vi "aotfController.vi"() -> ()   [LabVIEW 2024]
uses:
  <vilib>/Utility/error.llb/Trim Whitespace One-Sided.vi
  <vilib>/Instr/_visa.llb/VISA Configure Serial Port (Instr).vi
panel:
  in  "Stop Button":bool
  in  "Use":bool
  out "myaotf":refnum<k38>
  out "VISA out":refnum<visa-resource-name>="COM7"
  in  "VISA resource name":refnum<visa-resource-name>="COM7"
  out "module path":path=path "D:/Ortansia Multi Functional Controlling System/aotf/AOTFlabview.py"
  out "Py":refnum<k35>
  in  "fr":dbl=96.2
  in  "fg":dbl=114.86
  in  "ag":u32=10350
  in  "ar":u32=9820
  in  "ap":u32=100 max=110 step=10
  in  "ab":u32=16370
  in  "fb":dbl=137.52
  in  "red":bool
  in  "green":bool
  in  "blue":bool
  in  "purple":bool
  out "error out":errorcluster
  out "Info":string="BoardID serial\r\nSerial Number: 148B3A8606000025\r\n* dau en | dau en\r\n* dds a 0 0 | dds a 0 0\r\n* dds a 1 0 | dds a 1 0\r\n* dds a 2 0 | dds a 2 0\r\n* dds a 3 0 | dds a 3 0\r\n* dds a 4 0 | dds a 4 0\r\n* dds a 5 0 | dds a 5 0\r\n* dds a 6 0 | dds a 6 0\r\n* dds a 7 0 | dds a 7 0\r\n* OBIS S/N: S150224022\r\ndds a 0 0 | dds a 0 0\r\n* dds a 1 0 | dds a 1 0\r\n* dds a 2 0 | dds a 2 0\r\n* dds a 3 0 | dds a 3 0\r\n* dds a 4 0 | dds a 4 0\r\n* dds a 5 0 | dds a 5 0\r\n* dds a 6 0 | dds a 6 0\r\n* dds a 7 0 | dds a 7 0\r\n* dau dis | dau dis\r\n* res: Closed"
  # "ON/OFF"
  # "Frequency"
  # "Power"
  # "Limits"
  # "0~110 mW"
  # "0 ~ 16370 Pw"
  # "0 ~ 10350 Pw"
  # "0 ~ 9820 Pw"
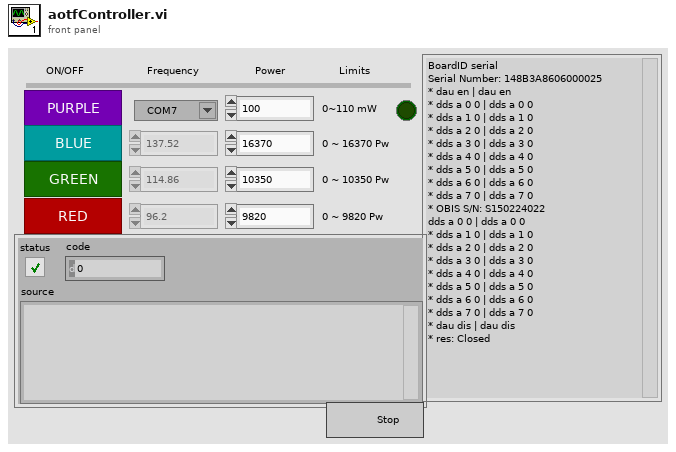
[diagram p1: front panel]
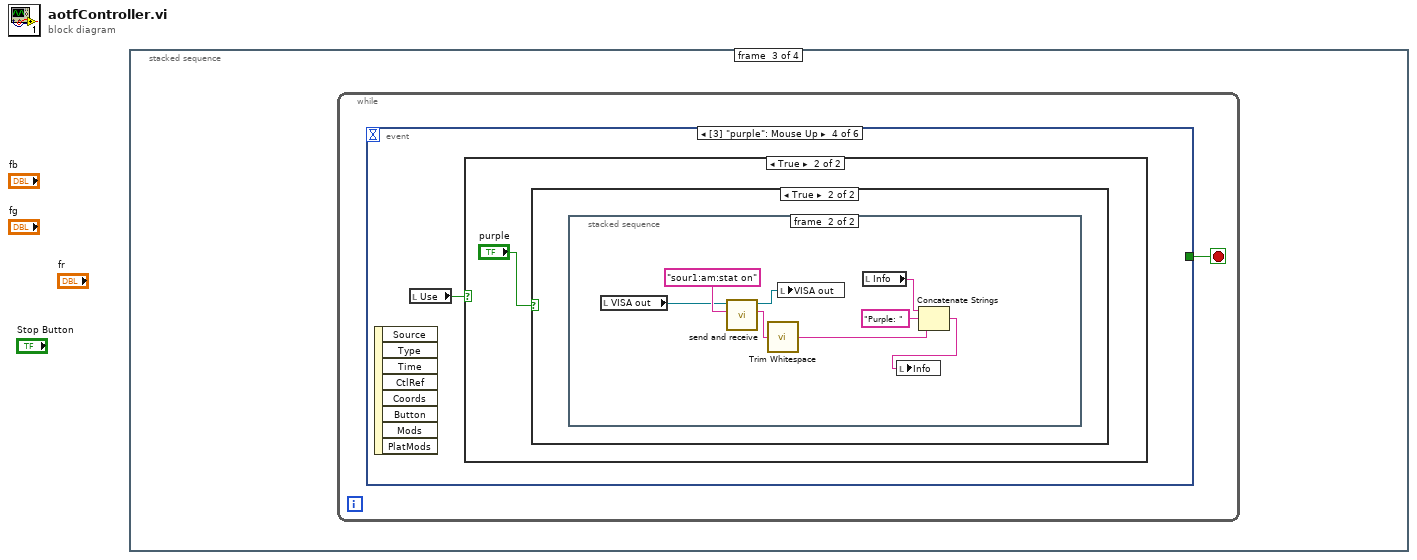
[diagram p0: block diagram]
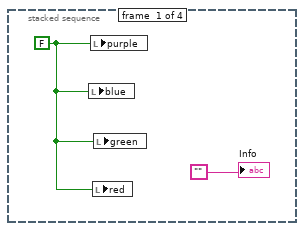
[diagram p2: hidden frame]
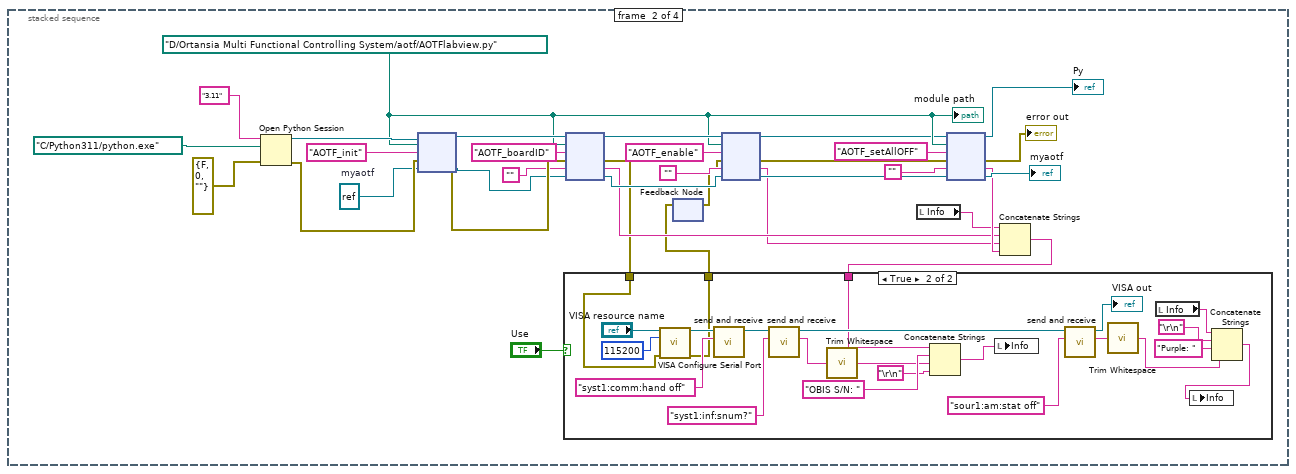
[diagram p3: hidden frame]
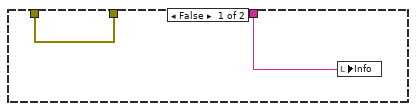
[diagram p4: hidden frame]
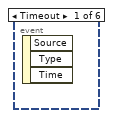
[diagram p5: hidden frame]
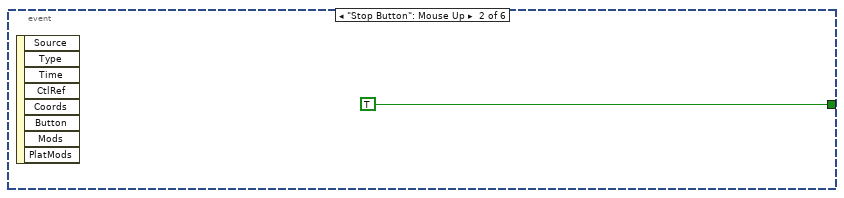
[diagram p6: hidden frame]
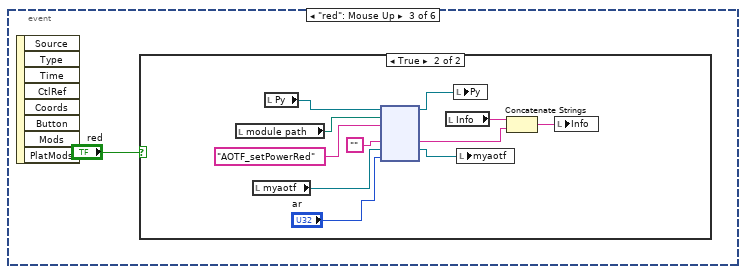
[diagram p7: hidden frame]
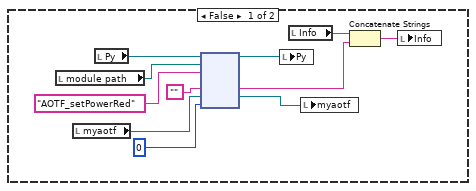
[diagram p8: hidden frame]
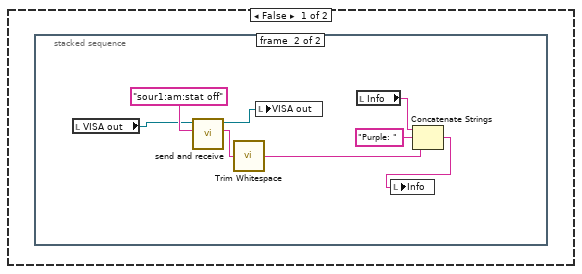
[diagram p10: hidden frame]
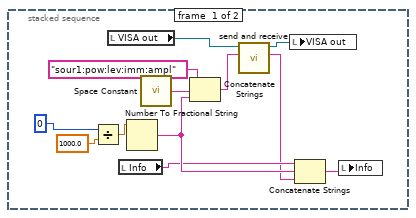
[diagram p11: hidden frame]
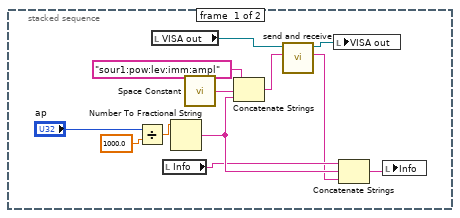
[diagram p12: hidden frame]
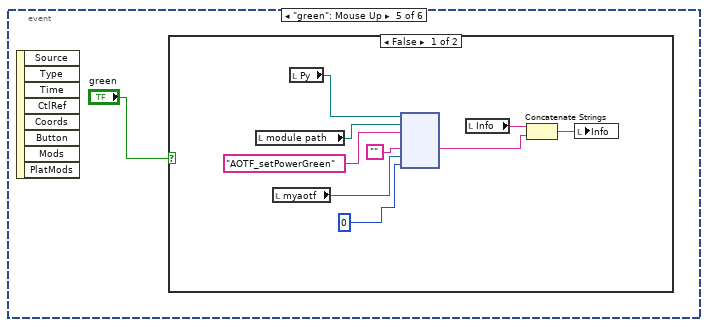
[diagram p13: hidden frame]
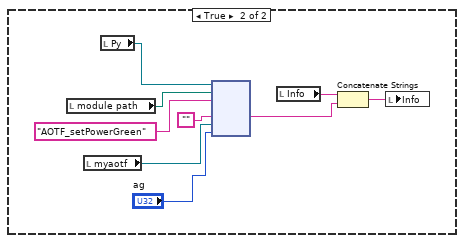
[diagram p14: hidden frame]
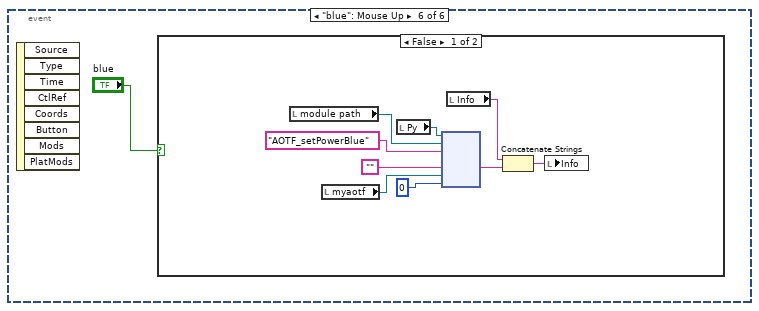
[diagram p15: hidden frame]
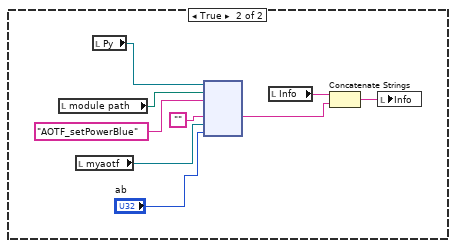
[diagram p16: hidden frame]
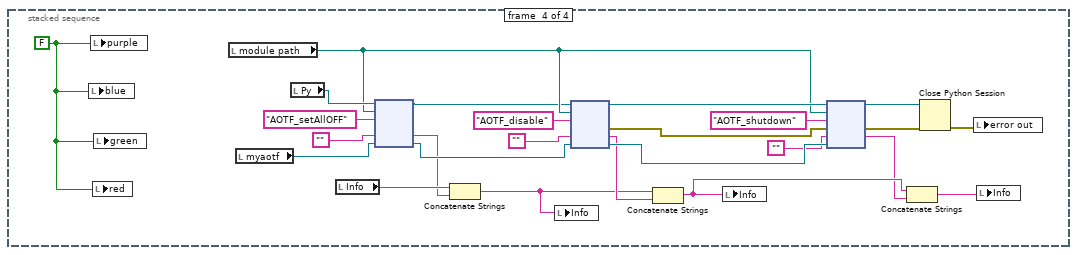
[diagram p17: hidden frame]
diagram:
  n1 = stacked-sequence {
    frame #0 {
      w1 = FALSE ("purple")
      n2 = local write "blue"(w1) -> ()
      n3 = local write "purple"(w1) -> ()
      n4 = local write "red"(w1) -> ()
      n5 = local write "green"(w1) -> ()
      "Info" <- ""
    }
    frame #1 {
      w29 = refnum<k38> refnum  # myaotf
      w14 = path "D:/Ortansia Multi Functional Controlling System/aotf/AOTFlabview.py" ("module path")
      n6 = Open Python Session(python version="3.11" ("Python version"), python path=path "C:/Python311/python.exe" ("Python path"), 3:errorcluster {"status"=FALSE, "code"=0, "source"=""} ("error in (no error)")) -> (session out=w27:refnum<k35>, error out=w35:errorcluster)
      n7 = node(w27, w14, "AOTF_init" ("function name"), w35, w29) -> (w30:refnum<k35>, w36:errorcluster, w33:refnum<k38>)  [unwired: 2 out]
      n8 = node(w30, w14, "AOTF_boardID" ("function name"), w36, "", w33) -> (w22:refnum<k35>, w8:errorcluster, w12:string, w21:refnum<k38>)  [unwired: 2 out]
      n9 = feedback #1() -> (w3:errorcluster)  [unwired: 1 in]
      n10 = node(w22, w14, "AOTF_enable" ("function name"), w3, "", w21) -> (w9:refnum<k35>, w16:errorcluster, w11:string, w18:refnum<k38>)  [unwired: 2 out]
      n11 = local read "Info"() -> (w7:string)
      n12 = node(w9, w14, "AOTF_setAllOFF" ("function name"), w16, "", w18) -> (→"Py":refnum<k35>, →"error out":errorcluster, w13:string, →"myaotf":refnum<k38>)  [unwired: 2 out]
      n13 = Concatenate Strings(w7, w12, w11, w13) -> (w6:string)
      n14 = case shown="True" "Use" {
        tunnel: w8 -> [w38 w47]
        tunnel: [w38 w46] -> w4
        tunnel: w6 -> [w37 w44]
        frame False {
          n15 = local write "Info"(w37) -> ()
        }
        frame True {
          n16 = call-poly "VISA Configure Serial Port"("VISA resource name"="VISA resource name", "baud rate (9600)"=u32 115200, "error in (no error)"=w47) -> ("VISA resource name out"=w58:refnum<visa-resource-name>, "error out"=w46:errorcluster)  [unwired: 11 in]
          n17 = call "send and receive.vi"("write to laser"="syst1:comm:hand off", "VISA resource name"=w58) -> ("VISA resource name out"=w56:refnum<visa-resource-name>)  [unwired: 8 in, 1 out]
          n18 = call "send and receive.vi"("write to laser"="syst1:inf:snum?", "VISA resource name"=w56) -> ("read from laser"=w50:string, "VISA resource name out"=w54:refnum<visa-resource-name>)  [unwired: 8 in]
          n19 = call <vilib>:"Trim Whitespace.vi"("string"=w50) -> ("trimmed string"=w48:string)  [unwired: 1 in]
          n20 = Concatenate Strings(w44, "OBIS S/N: ", w48, "\r\n") -> (w55:string)
          n21 = local write "Info"(w55) -> ()
          n22 = call "send and receive.vi"("write to laser"="sour1:am:stat off", "VISA resource name"=w54) -> ("read from laser"=w52:string, "VISA resource name out"=→"VISA out":refnum<visa-resource-name>)  [unwired: 8 in]
          n23 = call <vilib>:"Trim Whitespace.vi"("string"=w52) -> ("trimmed string"=w42:string)  [unwired: 1 in]
          n24 = local read "Info"() -> (w40:string)
          n25 = Concatenate Strings(w40, "\r\n", "Purple: " ("string"), w42) -> (w41:string)
          n26 = local write "Info"(w41) -> ()
        }
      }
      n27 = feedback-in #1(w4) -> ()
      "module path" <- w14
    }
    frame #2 {
      n28 = while {
        stop <- w62 stop-if-true
        n29 = event shown="[3] \"purple\": Mouse Up" {
          selector: _ -> [_ _ _ _ _ _]
          dyn-events: _ -> [_ _ _ _ _ _]
          timeout: _ -> [_ _ _ _ _ _]
          tunnel: [_ TRUE ("Stop Button") _ _ _ _] -> w62
          event Timeout {
            n30 = event-data() -> ()  [unwired: 1 in, 3 out]
          }
          event "Stop Button": Mouse Up {
            n31 = event-data() -> ()  [unwired: 1 in, 8 out]
          }
          event "red": Mouse Up {
            n32 = event-data() -> ()  [unwired: 1 in, 8 out]
            n33 = case shown="True" "red" {
              frame False {
                n34 = local read "module path"() -> (w74:path)
                n35 = local read "myaotf"() -> (w72:refnum<k38>)
                n36 = local read "Py"() -> (w75:refnum<k35>)
                n37 = node(w75, w74, "AOTF_setPowerRed" ("function name"), "", w72, u32 0 ("input parameter")) -> (w66:refnum<k35>, w69:string, w65:refnum<k38>)  [unwired: 2 in, 3 out]
                n38 = local write "Py"(w66) -> ()
                n39 = local read "Info"() -> (w70:string)
                n40 = local write "myaotf"(w65) -> ()
                n41 = Concatenate Strings(w70, w69) -> (w68:string)
                n42 = local write "Info"(w68) -> ()
              }
              frame True {
                n43 = local read "module path"() -> (w85:path)
                n44 = local read "myaotf"() -> (w83:refnum<k38>)
                n45 = local read "Py"() -> (w86:refnum<k35>)
                n46 = node(w86, w85, "AOTF_setPowerRed" ("function name"), "", w83, "ar") -> (w77:refnum<k35>, w79:string, w76:refnum<k38>)  [unwired: 2 in, 3 out]
                n47 = local read "Info"() -> (w80:string)
                n48 = local write "Py"(w77) -> ()
                n49 = local write "myaotf"(w76) -> ()
                n50 = Concatenate Strings(w80, w79) -> (w78:string)
                n51 = local write "Info"(w78) -> ()
              }
            }
          }
          event "purple": Mouse Up {
            n52 = event-data() -> ()  [unwired: 1 in, 8 out]
            n53 = local read "Use"() -> (w87:bool)
            n54 = case shown="True" w87 {
              frame False {
              }
              frame True {
                n55 = case shown="True" "purple" {
                  frame False {
                    n56 = stacked-sequence {
                      frame #0 {
                        n57 = Divide(x=0, y=1000.0) -> (x/y=w96:dbl)
                        n58 = local read "VISA out"() -> (w94:refnum<visa-resource-name>)
                        n59 = local read "Info"() -> (w93:string)
                        n60 = Number To Fractional String(number=w96) -> (F-format string=w95:string)  [unwired: 3 in]
                        n61 = call <vilib>:"Space Constant.vi"() -> ("String"=w99:string)
                        n62 = Concatenate Strings("sour1:pow:lev:imm:ampl", w99, w95) -> (w98:string)
                        n63 = call "send and receive.vi"("write to laser"=w98, "VISA resource name"=w94) -> ("read from laser"=w91:string, "VISA resource name out"=w92:refnum<visa-resource-name>)  [unwired: 8 in]
                        n64 = local write "VISA out"(w92) -> ()
                        n65 = Concatenate Strings(w93, w95, w91) -> (w90:string)
                        n66 = local write "Info"(w90) -> ()
                      }
                      frame #1 {
                        n67 = local read "VISA out"() -> (w102:refnum<visa-resource-name>)
                        n68 = call "send and receive.vi"("write to laser"="sour1:am:stat off", "VISA resource name"=w102) -> ("read from laser"=w108:string, "VISA resource name out"=w101:refnum<visa-resource-name>)  [unwired: 8 in]
                        n69 = call <vilib>:"Trim Whitespace.vi"("string"=w108) -> ("trimmed string"=w103:string)  [unwired: 1 in]
                        n70 = local write "VISA out"(w101) -> ()
                        n71 = local read "Info"() -> (w106:string)
                        n72 = Concatenate Strings(w106, "Purple: " ("string"), w103) -> (w105:string)
                        n73 = local write "Info"(w105) -> ()
                      }
                    }
                  }
                  frame True {
                    n74 = stacked-sequence {
                      frame #0 {
                        n75 = Divide(x="ap", y=1000.0) -> (x/y=w116:dbl)
                        n76 = local read "VISA out"() -> (w114:refnum<visa-resource-name>)
                        n77 = local read "Info"() -> (w112:string)
                        n78 = Number To Fractional String(number=w116) -> (F-format string=w115:string)  [unwired: 3 in]
                        n79 = call <vilib>:"Space Constant.vi"() -> ("String"=w119:string)
                        n80 = Concatenate Strings("sour1:pow:lev:imm:ampl", w119, w115) -> (w118:string)
                        n81 = call "send and receive.vi"("write to laser"=w118, "VISA resource name"=w114) -> ("read from laser"=w110:string, "VISA resource name out"=w111:refnum<visa-resource-name>)  [unwired: 8 in]
                        n82 = local write "VISA out"(w111) -> ()
                        n83 = Concatenate Strings(w112, w115, w110) -> (w109:string)
                        n84 = local write "Info"(w109) -> ()
                      }
                      frame #1 {
                        n85 = local read "VISA out"() -> (w121:refnum<visa-resource-name>)
                        n86 = call "send and receive.vi"("write to laser"="sour1:am:stat on", "VISA resource name"=w121) -> ("read from laser"=w128:string, "VISA resource name out"=w122:refnum<visa-resource-name>)  [unwired: 8 in]
                        n87 = call <vilib>:"Trim Whitespace.vi"("string"=w128) -> ("trimmed string"=w123:string)  [unwired: 1 in]
                        n88 = local write "VISA out"(w122) -> ()
                        n89 = local read "Info"() -> (w126:string)
                        n90 = Concatenate Strings(w126, "Purple: " ("string"), w123) -> (w125:string)
                        n91 = local write "Info"(w125) -> ()
                      }
                    }
                  }
                }
              }
            }
          }
          event "green": Mouse Up {
            n92 = event-data() -> ()  [unwired: 1 in, 8 out]
            n93 = case shown="False" "green" {
              frame False {
                n94 = local read "module path"() -> (w137:path)
                n95 = local read "myaotf"() -> (w135:refnum<k38>)
                n96 = local read "Py"() -> (w138:refnum<k35>)
                n97 = node(w138, w137, "AOTF_setPowerGreen" ("function name"), "", w135, u32 0 ("input parameter")) -> (w132:string)  [unwired: 3 in, 4 out]
                n98 = local read "Info"() -> (w133:string)
                n99 = Concatenate Strings(w133, w132) -> (w131:string)
                n100 = local write "Info"(w131) -> ()
              }
              frame True {
                n101 = local read "module path"() -> (w146:path)
                n102 = local read "myaotf"() -> (w144:refnum<k38>)
                n103 = local read "Py"() -> (w147:refnum<k35>)
                n104 = node(w147, w146, "AOTF_setPowerGreen" ("function name"), "", w144, "ag") -> (w141:string)  [unwired: 3 in, 4 out]
                n105 = local read "Info"() -> (w142:string)
                n106 = Concatenate Strings(w142, w141) -> (w140:string)
                n107 = local write "Info"(w140) -> ()
              }
            }
          }
          event "blue": Mouse Up {
            n108 = event-data() -> ()  [unwired: 1 in, 8 out]
            n109 = case shown="False" "blue" {
              frame False {
                n110 = local read "module path"() -> (w156:path)
                n111 = local read "myaotf"() -> (w155:refnum<k38>)
                n112 = local read "Py"() -> (w157:refnum<k35>)
                n113 = node(w157, w156, "AOTF_setPowerBlue" ("function name"), "", w155, u32 0 ("input parameter")) -> (w153:string)  [unwired: 3 in, 4 out]
                n114 = local read "Info"() -> (w154:string)
                n115 = Concatenate Strings(w154, w153) -> (w152:string)
                n116 = local write "Info"(w152) -> ()
              }
              frame True {
                n117 = local read "module path"() -> (w165:path)
                n118 = local read "myaotf"() -> (w163:refnum<k38>)
                n119 = local read "Py"() -> (w166:refnum<k35>)
                n120 = node(w166, w165, "AOTF_setPowerBlue" ("function name"), "", w163, "ab") -> (w160:string)  [unwired: 3 in, 4 out]
                n121 = local read "Info"() -> (w161:string)
                n122 = Concatenate Strings(w161, w160) -> (w159:string)
                n123 = local write "Info"(w159) -> ()
              }
            }
          }
        }
      }
    }
    frame #3 {
      w177 = FALSE ("purple")
      n124 = local write "blue"(w177) -> ()
      n125 = local write "purple"(w177) -> ()
      n126 = local write "red"(w177) -> ()
      n127 = local write "green"(w177) -> ()
      n128 = local read "module path"() -> (w172:path)
      n129 = local read "myaotf"() -> (w176:refnum<k38>)
      n130 = local read "Py"() -> (w175:refnum<k35>)
      n131 = local read "Info"() -> (w169:string)
      n132 = node(w175, w172, "AOTF_setAllOFF" ("function name"), "", w176) -> (w171:refnum<k35>, w167:string, w170:refnum<k38>)  [unwired: 1 in, 3 out]
      n133 = Concatenate Strings(w169, w167) -> (w168:string)
      n134 = local write "Info"(w168) -> ()
      n135 = node(w171, w172, "AOTF_disable" ("function name"), "", w170) -> (w183:refnum<k35>, w185:errorcluster, w187:string, w188:refnum<k38>)  [unwired: 1 in, 2 out]
      n136 = Concatenate Strings(w168, w187) -> (w191:string)
      n137 = local write "Info"(w191) -> ()
      n138 = node(w183, w172, "AOTF_shutdown" ("function name"), w185, "", w188) -> (w180:refnum<k35>, w181:errorcluster, w190:string)  [unwired: 1 in, 2 out]
      n139 = Concatenate Strings(w191, w190) -> (w189:string)
      n140 = Close Python Session(session in=w180, error in=w181) -> (11:w178:errorcluster)
      n141 = local write "error out"(w178) -> ()
      n142 = local write "Info"(w189) -> ()
    }
  }
